vi "Create Value - 1D Array Double.vi"(8 "error in (no error)":errorcluster, 9 "Create as 1D Array?":bool=TRUE, 10 "1D Numeric":dbl[](array[numeric])) -> (0 "error out":errorcluster, 3 "JSON Tree":variant)   [LabVIEW 2013, in "i3-json.lvlib"]
uses:
  i3-json.lvlib
  JSON Types/JSON Type.ctl
  JSON Types/JSON Compatible Type.ctl
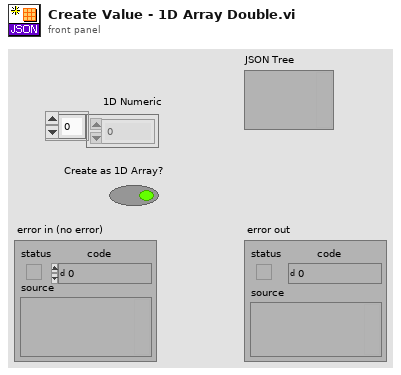
[diagram p1: front panel]
types:
  T1 = typedef "i3-json.lvlib/JSON Compatible Type.ctl" = enum16{"1D Double Array", "1D String Array", "1D Boolean Array", "Unknown"}
  T2 = typedef "i3-json.lvlib/JSON Type.ctl" = enum8{"JSON Compatible", "JSON Array", "JSON Object", "JSON Null", "Double", "String", "Boolean", "Unknown", "Data JSON string"}
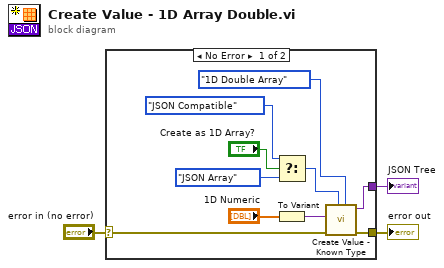
[diagram p0: block diagram]
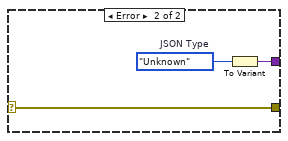
[diagram p2: hidden frame]
diagram:
  n1 = case shown="No Error" "error in (no error)" {
    selector: "error in (no error)" -> [w12 w14]
    tunnel: [w11 w14] -> w2
    tunnel: [w13 w15] -> w1
    frame No Error {
      n2 = Select(t=JSON_Type."JSON Compatible" ("JSON Type"), s="Create as 1D Array?", f=JSON_Type."JSON Array" ("JSON Type")) -> (s? t:f=w6:T2)
      n3 = To Variant(anything="1D Numeric") -> (Variant=w9:variant)
      n4 = call "Create Value - Known Type.vi"("JSON Compatible Type"=JSON_Compatible_Type."1D Double Array", "JSON Type"=w6, "error in (no error)"=w12, "Value"=w9) -> ("error out"=w11:errorcluster, "JSON Tree"=w13:variant)  [unwired: 6 in]
    }
    frame Error {
      w16 = JSON_Type."Unknown"  # JSON Type
      n5 = To Variant(anything=w16) -> (Variant=w15:variant)
    }
  }
  "JSON Tree" <- w1
  "error out" <- w2
